vi "ControllingMotor_Class_1.vi"() -> ()   [LabVIEW 2015]
panel:
  out "Current Speed 2":dbl(knob)=0.4485598347338502 scale=-1.0..1.0
  in  "Set Speed 2":dbl(knob)=0.44855983482262074 scale=-1.0..1.0
  in  "Scale":dbl=0.5
  out "Current Speed":dbl(knob)=0.4485598347338502 scale=-1.0..1.0
  in  "Hard Stop":bool
  in  "standby":bool
  in  "Set Speed":dbl(knob)=0.44855983482262074 scale=-1.0..1.0
  # "Wheel Controls"
  # "Wheel Controls"
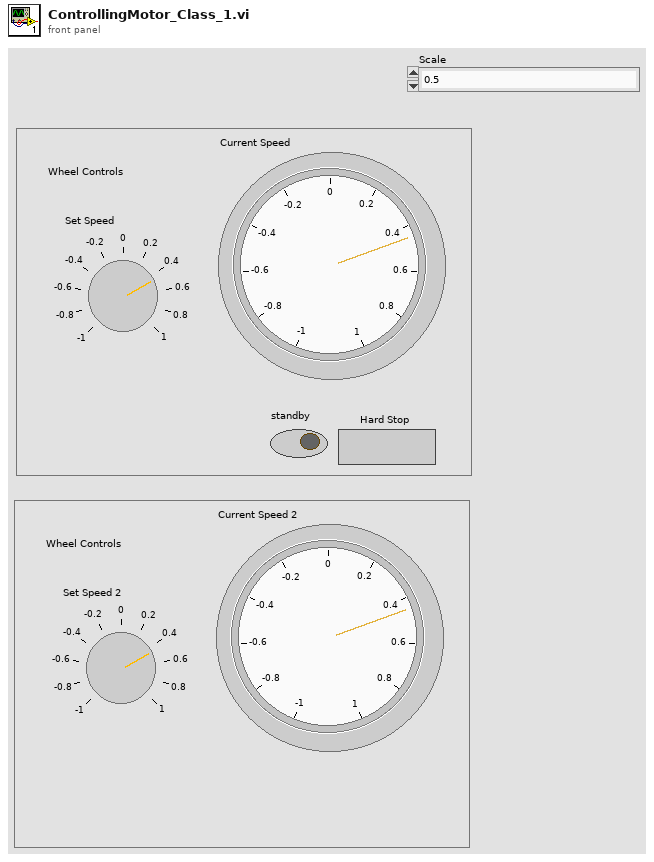
[diagram p1: front panel]
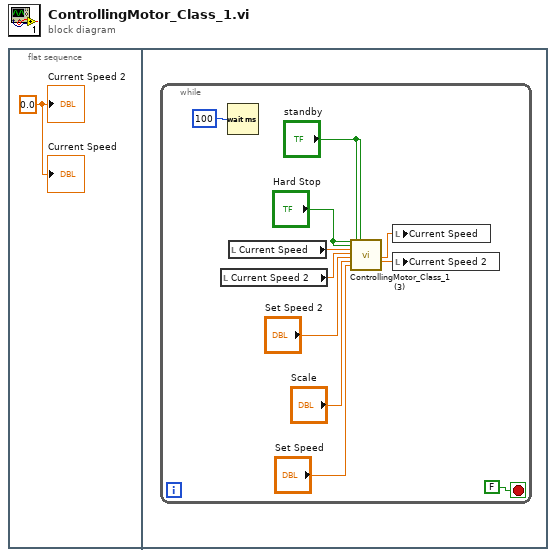
[diagram p0: block diagram]
diagram:
  n1 = flat-sequence {
    frame #0 {
      w1 = 0.0 ("Current Speed")
      "Current Speed" <- w1
      "Current Speed 2" <- w1
    }
    frame #1 {
      n2 = while {
        stop <- FALSE stop-if-true
        n3 = local read "Current Speed 2"() -> (w4:dbl)
        n4 = Wait (ms)(milliseconds to wait=u32 100) -> ()  [unwired: 1 out]
        n5 = local read "Current Speed"() -> (w7:dbl)
        n6 = call "ControllingMotor_Class_1 (3).vi"("Hard Stop"="Hard Stop", "Hard Stop 2"="Hard Stop", "Current Speed"=w7, "Current Speed 2"=w4, "Set Speed 2"="Set Speed 2", "Scale"="Scale", "Set Speed"="Set Speed", "standby"="standby", "standby 2"="standby") -> ("New Speed 2"=w11:dbl, "New Speed"=w8:dbl)  [unwired: 5 in, 12 out]
        n7 = local write "Current Speed"(w11) -> ()
        n8 = local write "Current Speed 2"(w8) -> ()
      }
    }
  }
